vi "Move to whole rev.vi"(5 "resource in":refnum<k21>="Axis 8", 6 "Default Motor Parameters":T1={"position"=10000.0, "velocity"=10000.0, "acceleration"=100000.0, "deceleration"=100000.0, "accel. jerk"=1000000.0, "decel. jerk"=1000000.0}, 7 "Mode":enum16{"ABS Pos Move", "REL Pos Move"}(ring), 8 "error in (no error)":errorcluster, 9 "cts per rev":dbl=1000.0 format="%#_13g", 10 "# whole revs":dbl=5.0, 11 "Queue in":refnum<queue>) -> (0 "error out":errorcluster, 3 "Queue out":refnum<queue>)   [LabVIEW 2014]
uses:
  support/Message Queue/Message Cluster.ctl
  EMC API/EMC_Typedef_Motor_Parameters.ctl
  Typedef/Typedef_Motor_Message.ctl
  <vilib>/Motion/Express/_s/nimc.ex.read.readTrajectoryData.axis.vi
  <vilib>/Motion/BlockNode/FB.NIMotion.xnode
  support/Message Queue/Message Queue.lvlib
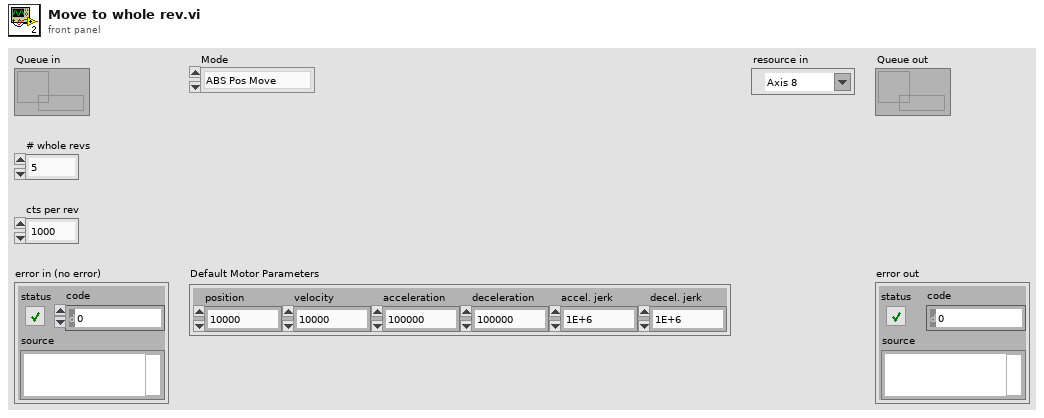
[diagram p1: front panel]
types:
  T1 = typedef "EMC_Typedef_Motor_Parameters.ctl" = cluster{"position":dbl, "velocity":dbl, "acceleration":dbl, "deceleration":dbl, "accel. jerk":dbl, "decel. jerk":dbl}
  T2 = typedef "Typedef_Motor_Message.ctl" = cluster{"Axis":refnum<k21>, "Motion Parameters":T1}
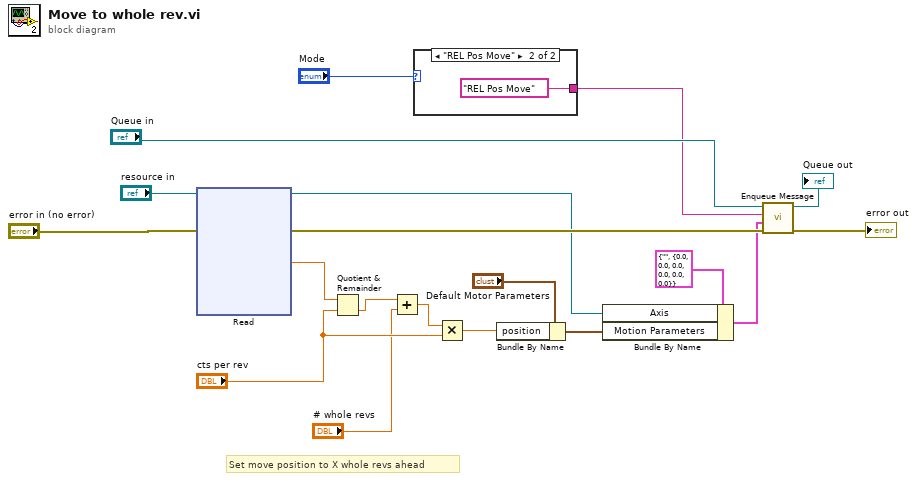
[diagram p0: block diagram]
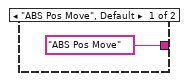
[diagram p2: hidden frame]
diagram:
  # "Set move position to X whole revs ahead"
  n1 = xnode ("Read")("resource"="resource in", "error in"="error in (no error)") -> ("commanded position"=w6:dbl, "resource out"=w11:refnum<k21>, "error out"=w15:errorcluster)  [unwired: 2 out]
  n2 = Quotient & Remainder(x=w6, y="cts per rev") -> (floor(x/y)=w7:dbl)  [unwired: 1 out]
  n3 = Add(x=w7, y="# whole revs") -> (x+y=w8:dbl)
  n4 = case shown="\"REL Pos Move\"" "Mode" {
    tunnel: ["ABS Pos Move" "REL Pos Move"] -> w3
    frame "ABS Pos Move", Default {
    }
    frame "REL Pos Move" {
    }
  }
  n5 = Multiply(x=w8, y="cts per rev") -> (x*y=w18:dbl)
  n6 = Bundle By Name(cluster="Default Motor Parameters", "position"=w18) -> (w12:T1)
  n7 = Bundle By Name(cluster=T2 {"Axis"="", "Motion Parameters"={"position"=0.0, "velocity"=0.0, "acceleration"=0.0, "deceleration"=0.0, "accel. jerk"=0.0, "decel. jerk"=0.0}} ("Motor_Message"), "Axis"=w11, "Motion Parameters"=w12) -> (w10:T2)
  n8 = call "Enqueue Message.vi"("error in (no error)"=w15, "Message Data"=w10, "Message"=w3, "Message Queue"="Queue in") -> ("error out"=→"error out":errorcluster, "dup Message Queue"=→"Queue out":refnum<queue>)  [unwired: 6 in]
